vi "WaitForTrigger.vi"(8 "Error In":errorcluster, 9 "Timeout (sec)":dbl, 10 "Line (1-8)":u8=1 min=1 max=8 step=1, 11 "Keithley 2602 In":refnum<visa-resource-name>) -> (0 "Error Out":errorcluster, 2 "Trigger Detected?":bool, 3 "Keithley 2602 Out":refnum<visa-resource-name>)   [LabVIEW 2012, in "Keithley-2602.lvlib"]
uses:
  Keithley-2602.lvlib
panel:
  out "Output":string
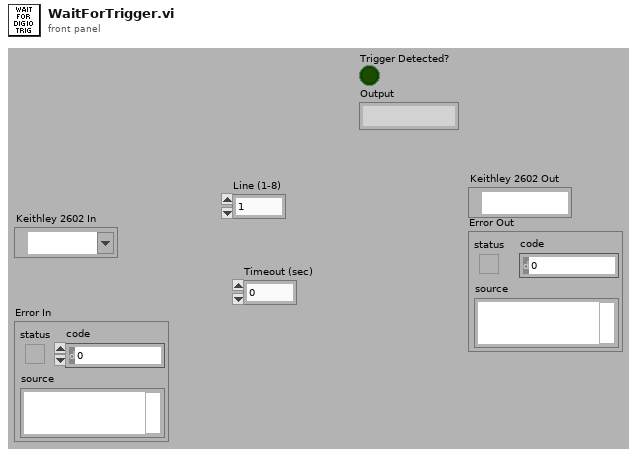
[diagram p1: front panel]
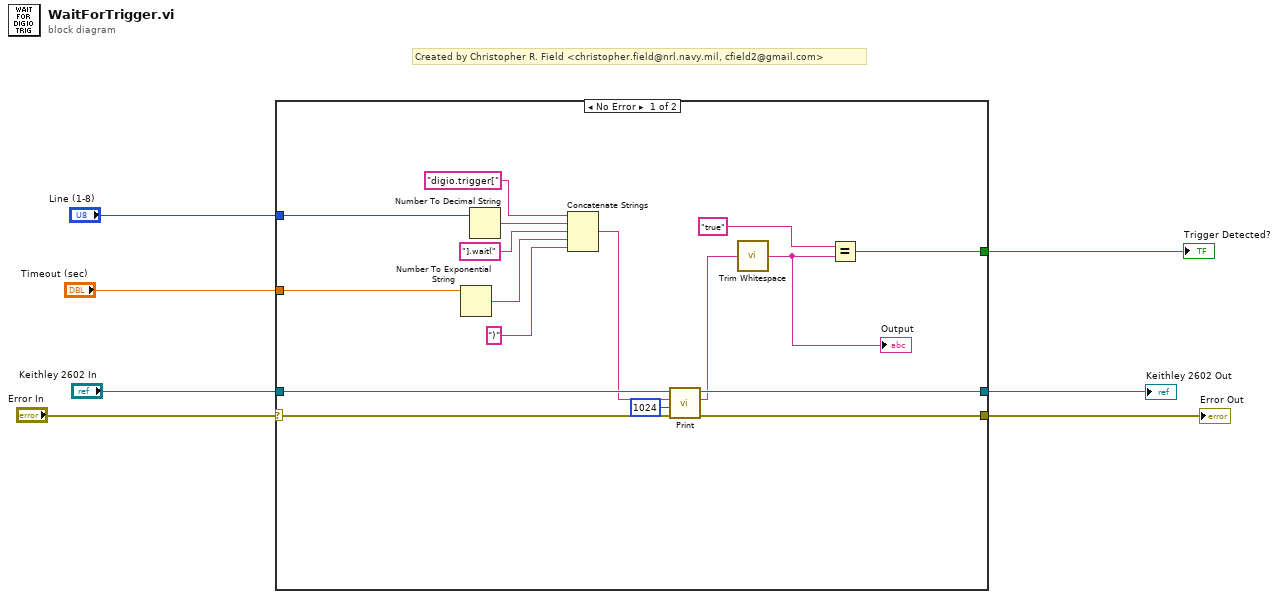
[diagram p0: block diagram]
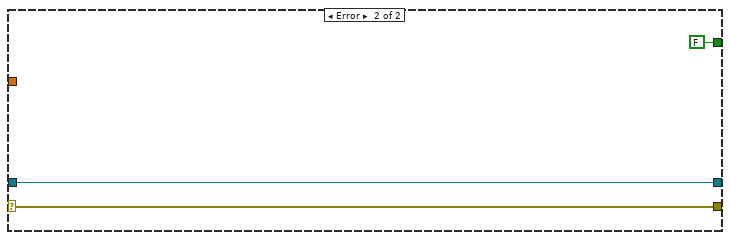
[diagram p2: hidden frame]
diagram:
  # "Created by Christopher R. Field <christopher.field@nrl.navy.mil, cfield2@gmail.com>"
  n1 = case shown="No Error" "Error In" {
    selector: "Error In" -> [w10 w26]
    tunnel: "Line (1-8)" -> [w24 _]
    tunnel: "Timeout (sec)" -> [w20 _]
    tunnel: "Keithley 2602 In" -> [w17 w27]
    tunnel: [w15 w27] -> w4
    tunnel: [w14 w26] -> w3
    tunnel: [w11 FALSE] -> w2
    frame No Error {
      n2 = Number To Exponential String(number=w20) -> (E-format string=w19:string)  [unwired: 3 in]
      n3 = Number To Decimal String(number=w24) -> (decimal integer string=w22:string)  [unwired: 1 in]
      n4 = Concatenate Strings("digio.trigger[", w22, "].wait(", w19, ")" ("string")) -> (w16:string)
      n5 = call "Print.vi"("Error In"=w10, "Byte Count"=u32 1024, "Attribute"=w16, "Kiethley 2602 In"=w17) -> ("Error Out"=w14:errorcluster, "Output"=w9:string, "Keithley 2602 Out"=w15:refnum<visa-resource-name>)  [unwired: 5 in]
      n6 = call <vilib>:"Trim Whitespace.vi"("string"=w9) -> ("trimmed string"=w8:string)  [unwired: 1 in]
      "Output" <- w8
      n7 = Equal?(x="true", y=w8) -> (x = y?=w11:bool)
    }
    frame Error {
    }
  }
  "Keithley 2602 Out" <- w4
  "Error Out" <- w3
  "Trigger Detected?" <- w2
